vi "RPC Method Invoke.vi"(8 "error in (no error)":errorcluster, 11 "OOP Server in":refnum<class "OOP Query Server.lvclass">) -> (0 "error out":errorcluster)   [LabVIEW 2019, in "OOP Query Server.lvlib" / "OOP Query Server.lvclass"]
uses:
  OOP Query Server.lvclass
  OOP Query Server.lvclass/OOP Query Server.ctl
  RPC Messages/InvokeResponse/InvokeResponse_Data.ctl
  typeDefs/Server Internal Data.ctl
  OOP Server/Class/OOP Server.lvclass
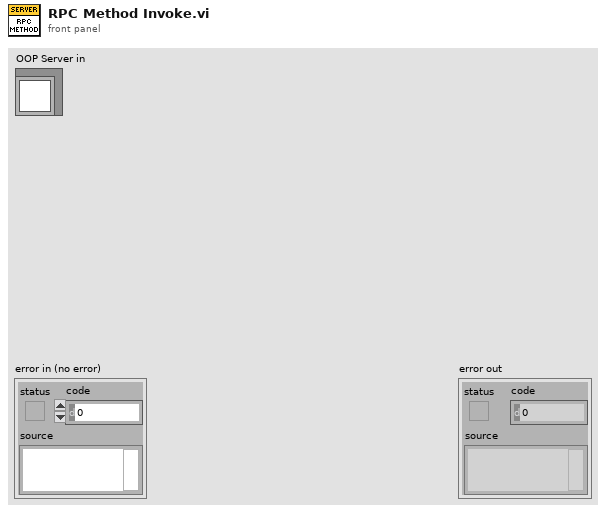
[diagram p1: front panel]
types:
  T1 = typedef "OOP Query Server.lvlib/OOP Query Server.lvclass/InvokeResponse_Data.ctl" = cluster{"status":i32}
  T2 = typedef "OOP Query Server.lvlib/OOP Query Server.lvclass/Server Internal Data.ctl" = cluster{"Command":string, "Data":variant}
  T3 = typedef "OOP Query Server.lvlib/OOP Query Server.lvclass/Server Internal UEs.ctl" = cluster{"Invoke Internal UE":refnum<user-event>, "Query Internal UE":refnum<user-event>, "Register Internal UE":refnum<user-event>}
  T4 = typedef "OOP Query Server.lvlib/OOP Query Server.lvclass/Server gRPC UEs.ctl" = cluster{"Invoke gRPC UE":refnum<user-event>, "Query gRPC UE":refnum<user-event>, "Register gRPC UE":refnum<user-event>}
  T5 = typedef "OOP Query Server.lvlib/gprc-lvsupport.lvlib/grpcId.ctl" = u64
  T6 = typedef "OOP Server.lvlib/OOP Server.lvclass/InvokeRequest_Data.ctl" = cluster{"command":string, "parameter":string}
  T7 = typedef "gprc-lvsupport.lvlib/grpcId.ctl" = u64
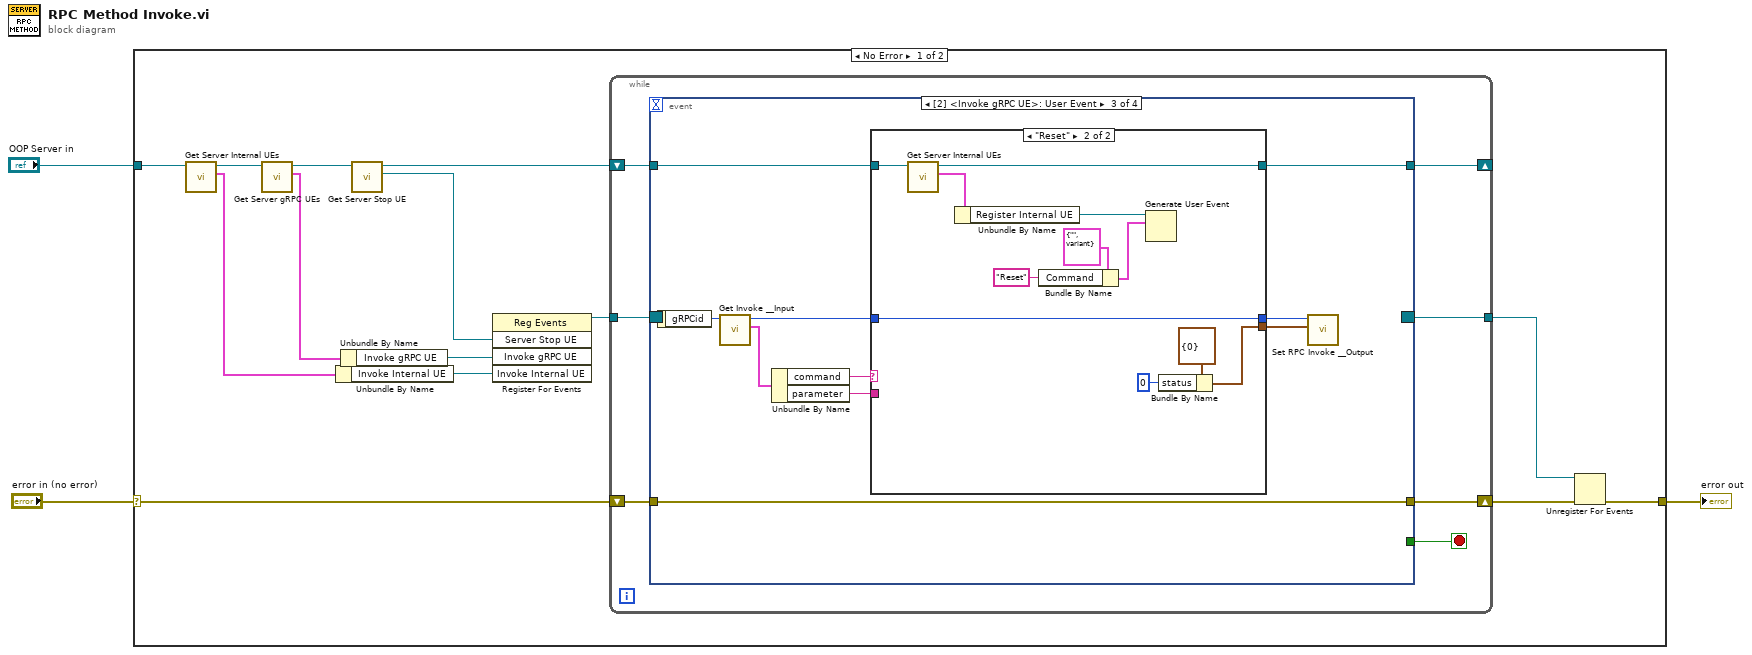
[diagram p0: block diagram]
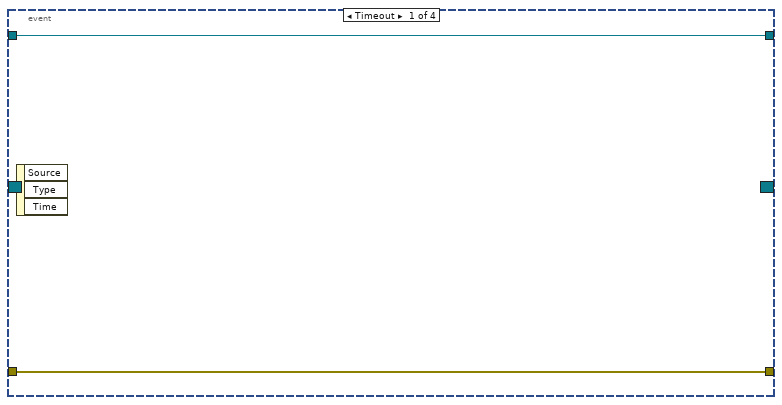
[diagram p2: hidden frame]
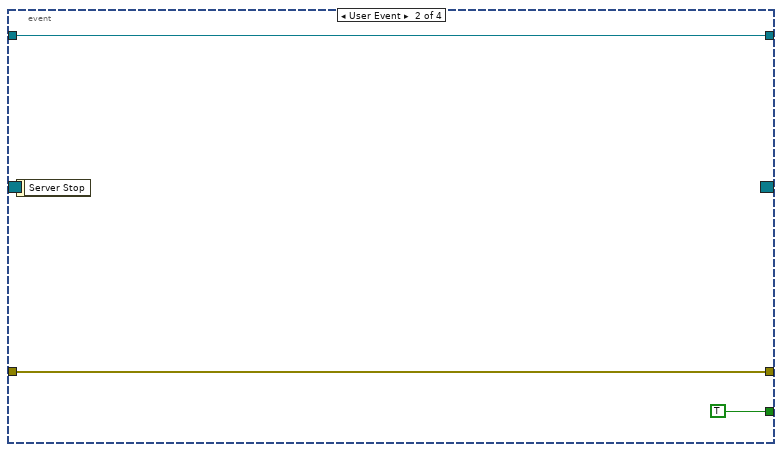
[diagram p3: hidden frame]
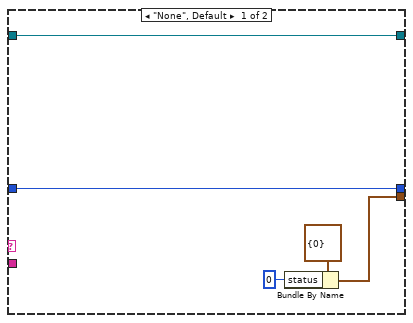
[diagram p4: hidden frame]
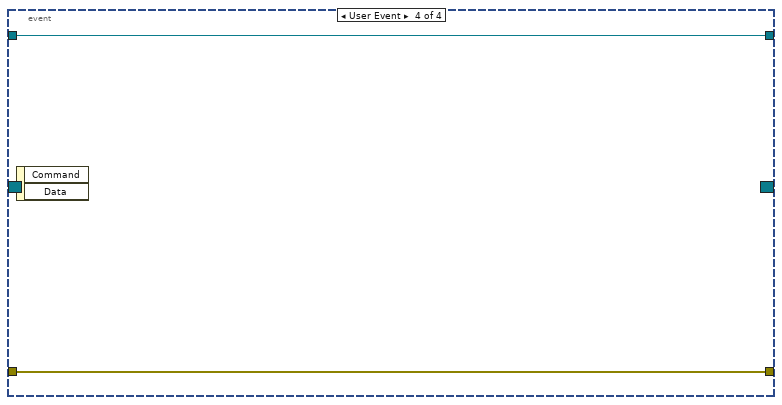
[diagram p5: hidden frame]
diagram:
  n1 = case shown="No Error" "error in (no error)" {
    selector: "error in (no error)" -> [w12 w58]
    tunnel: [w10 w58] -> w2
    tunnel: "OOP Server in" -> [w14 _]
    frame No Error {
      n2 = call "Get Server Internal UEs.vi"("OOP Server in"=w14) -> ("Server Internal UEs"=w6:T3, "OOP Server out"=w13:refnum<class "OOP Query Server.lvclass">)  [unwired: 9 in]
      n3 = call "Get Server gRPC UEs.vi"("OOP Server in"=w13) -> ("Server gRPC UEs"=w8:T4, "OOP Server out"=w17:refnum<class "OOP Query Server.lvclass">)  [unwired: 9 in]
      n4 = Unbundle By Name ("Unbundle Internal UE")(w6) -> ("Invoke Internal UE"=w5:refnum<user-event>)
      n5 = Unbundle By Name ("Unbundle gRPC UE")(w8) -> ("Invoke gRPC UE"=w7:refnum<user-event>)
      n6 = call "Get Server Stop UE.vi"("OOP Server in"=w17) -> ("Server Stop UE"=w16:refnum<user-event>, "OOP Server out"=w4:refnum<class "OOP Query Server.lvclass">)  [unwired: 9 in]
      n7 = register-events(w16, w7, w5) -> (reference out=w15:refnum<event-registration>)  [unwired: 2 in, 1 out]
      n8 = while {
        tunnel: w15 -> [w24]
        tunnel: [w20] -> w9
        shift-right: [w21] -> w11
        shift-left: w12 -> [w22]
        shift-right: [w18] -> _
        shift-left: w4 -> [w19]
        stop <- w23 stop-if-true
        n9 = event "RPC Method Event Structure" shown="[2] <Invoke gRPC UE>: User Event" {
          selector: w24 -> [_ _ _ _]
          dyn-events: [_ _ _ _] -> w20
          timeout: _ -> [_ _ _ _]
          tunnel: [_ TRUE _ _] -> w23
          tunnel: w22 -> [w26 w28 w30 w56]
          tunnel: [w26 w28 w30 w56] -> w21
          tunnel: w19 -> [w25 w27 w35 w57]
          tunnel: [w25 w27 w34 w57] -> w18
          event Timeout {
            n10 = event-data() -> ()  [unwired: 1 in, 3 out]
          }
          event User Event {
            n11 = event-data() -> ()  [unwired: 1 in, 1 out]
          }
          event User Event {
            n12 = event-data() -> ("gRPCid"=w39:T5)  [unwired: 1 in]
            n13 = call "Get Invoke __Input.vi"("gRPCid"=w39) -> ("Message Data"=w38:T6, "gRPCid out"=w33:T7)  [unwired: 8 in, 1 out]
            n14 = Unbundle By Name(w38) -> ("command"=w37:string, "parameter"=w36:string)
            n15 = case shown="\"Reset\"" w37 {
              tunnel: w36 -> [_ _]
              tunnel: w35 -> [w44 w55]
              tunnel: [w44 w49] -> w34
              tunnel: w33 -> [w43 w48]
              tunnel: [w43 w48] -> w32
              tunnel: [w40 w45] -> w31
              frame "None", Default {
                n16 = Bundle By Name(cluster=T1 {"status"=0} ("Message Data"), "status"=0) -> (w40:T1)
              }
              frame "Reset" {
                n17 = call "Get Server Internal UEs.vi"("OOP Server in"=w55) -> ("Server Internal UEs"=w54:T3, "OOP Server out"=w49:refnum<class "OOP Query Server.lvclass">)  [unwired: 9 in]
                n18 = Unbundle By Name(w54) -> ("Register Internal UE"=w53:refnum<user-event>)
                n19 = Bundle By Name(cluster=T2 {"Command"="", "Data"=variant} ("event data"), "Command"="Reset") -> (w51:T2)
                n20 = Generate User Event(user event=w53, event data cluster=w51) -> ()  [unwired: 2 in, 2 out]
                n21 = Bundle By Name(cluster=T1 {"status"=0} ("Message Data"), "status"=0) -> (w45:T1)
              }
            }
            n22 = call "Set RPC Invoke __Output.vi"("Message Data"=w31, "gRPCid in"=w32) -> ()  [unwired: 9 in, 1 out]
          }
          event User Event {
            n23 = event-data() -> ()  [unwired: 1 in, 2 out]
          }
        }
      }
      n24 = Unregister For Events(event registration refnum=w9, error in=w11) -> (error out=w10:errorcluster)
    }
    frame Error {
    }
  }
  "error out" <- w2
